vi "JYGetSlits.vi"(0 "MonoRefNum IN":refnum<k7>, 1 "UniqueID":string, 2 "Slit":u16(ring) items=["Front Entrance", "Side Entrance", "Front Exit", "Side Exit", "First Intermediate", "Second Intermediate"], 5 "error in (no error)":errorcluster) -> (12 "Units":string, 14 "MonoRefNum Out":refnum<k7>, 15 "Slit Width":dbl, 19 "error out":errorcluster)   [LabVIEW 2009]
doc: "JYGetSlits.vi\n\nUse this VI to get the current slit widths and the current default\nunits.\n\nInputs\nMonoRefNum In - LabView automation refnum for the current mono\nInput Error Cluster\n\nOutputs\nMonoRefNum Out - LabView automation refnum for the current mono\nF_En - double; current width of Front Entrance Slit\nF_Ex - double; current width of Front Exit Slit\nS_En - double; current width of Side Entrance Slit\nS_Ex - double; current width of Side Exit Slit\nUnits - string; slit width units\nOutput Error Cluster"
panel:
  out "UseUniqueID":bool
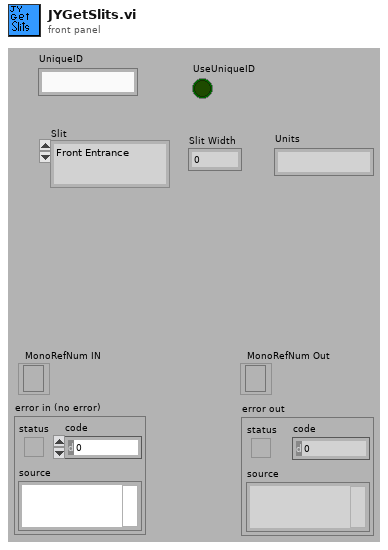
[diagram p1: front panel]
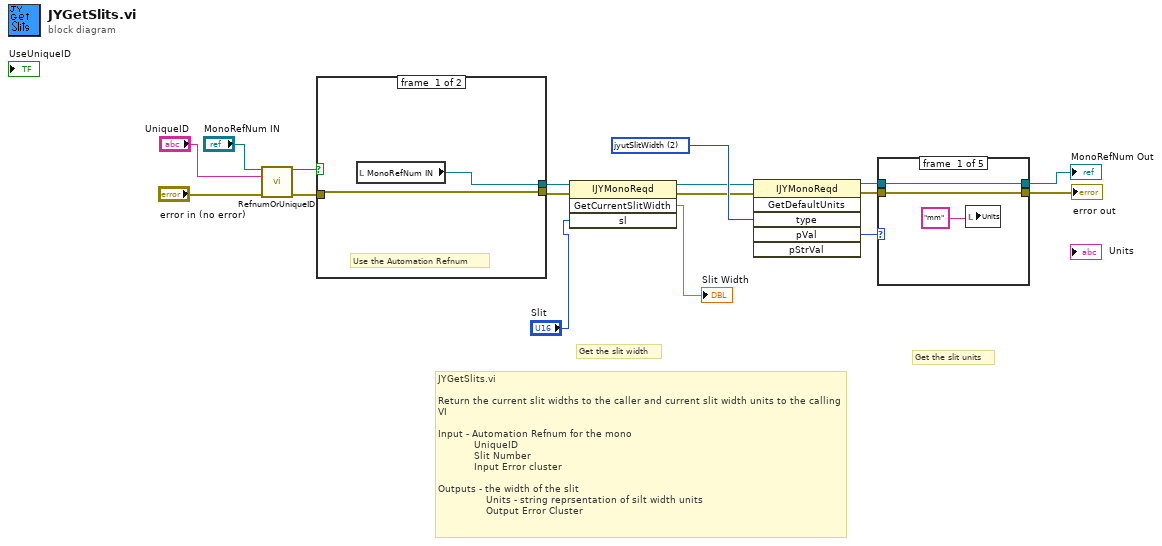
[diagram p0: block diagram]
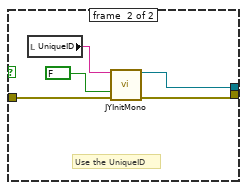
[diagram p2: hidden frame]
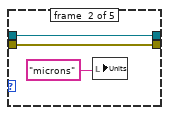
[diagram p3: hidden frame]
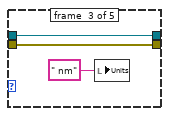
[diagram p4: hidden frame]
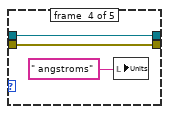
[diagram p5: hidden frame]
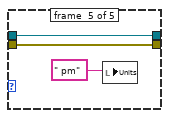
[diagram p6: hidden frame]
diagram:
  w16 = 2 items=["jyutUndefined", "jyutWavelength", "jyutSlitWidth", "jyutTime", "jyutTemperature", "jyutDataUnits", "jyutSpatial", "jyutTotalTypesPlusOne"] ("type")
  # "Get the slit units"
  # "Get the slit width"
  # "JYGetSlits.vi\n\nReturn the current slit widths to the caller and current slit width units to the calling VI\n\nInput - Automation Refnum for the mono\n            UniqueID\n            Slit Number\n            Input Error cluster\n\nOutputs - the width of the slit\n                Units - string reprsentation of silt width units\n                Output Error Cluster"
  n1 = call "RefnumOrUniqueID.vi"("Refnum IN"="MonoRefNum IN", "String in"="UniqueID", "error in (no error)"="error in (no error)") -> ("UseUniqueID"=w8:bool, "error out"=w5:errorcluster)  [unwired: 11 out]
  n2 = case shown="False" w8 {
    tunnel: [w19 w22] -> w7
    tunnel: w5 -> [w18 w21]
    tunnel: [w18 w20] -> w4
    frame #0 {
      # "Use the Automation Refnum"
      n3 = local read "MonoRefNum IN"() -> (w19:refnum<k7>)
    }
    frame #1 {
      # "Use the UniqueID"
      n4 = local read "UniqueID"() -> (w24:string)
      n5 = call "JYInitMono.vi"("Unique ID"=w24, "Force Init"=FALSE, "error in (no error)"=w21) -> ("Mono RefNum out"=w22:refnum<k7>, "error out"=w20:errorcluster)  [unwired: 1 in, 10 out]
    }
  }
  n6 = invoke class="IJYMonoReqd" method="GetCurrentSlitWidth"(reference=w7, error in=w4, "sl"="Slit") -> (reference out=w3:refnum<k7>, error out=w2:errorcluster, "GetCurrentSlitWidth"=→"Slit Width":dbl)  [unwired: 1 in, 1 out]
  n7 = invoke class="IJYMonoReqd" method="GetDefaultUnits"(reference=w3, error in=w2, "type"=w16) -> (reference out=w14:refnum<k7>, error out=w12:errorcluster, "pVal"=w15:i32)  [unwired: 3 in, 3 out]
  n8 = case shown="1, Default" w15 {
    tunnel: w14 -> [w26 w29 w32 w35 w38]
    tunnel: [w26 w29 w32 w35 w38] -> w13
    tunnel: w12 -> [w25 w28 w31 w34 w37]
    tunnel: [w25 w28 w31 w34 w37] -> w11
    frame #0 {
      n9 = local write "Units"("mm") -> ()
    }
    frame #1 {
      n10 = local write "Units"("microns") -> ()
    }
    frame #2 {
      n11 = local write "Units"(" nm") -> ()
    }
    frame #3 {
      n12 = local write "Units"(" angstroms") -> ()
    }
    frame #4 {
      n13 = local write "Units"(" pm") -> ()
    }
  }
  "MonoRefNum Out" <- w13
  "error out" <- w11
